vi "get default pixel clock.vi"(8 "error in (no error)":errorcluster, 11 "Thorcam in":refnum<class "Thorcam.lvclass">) -> (0 "error out":errorcluster, 1 "pixel clock":dbl[unit], 3 "Thorcam out":refnum<class "Thorcam.lvclass">)   [LabVIEW 2012, in "Thorcam.lvclass"]
uses:
  Thorcam.lvclass
  Thorcam.lvclass/Thorcam.ctl
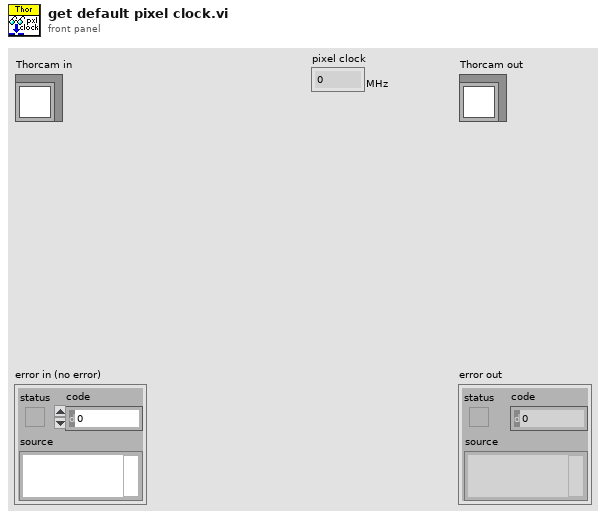
[diagram p1: front panel]
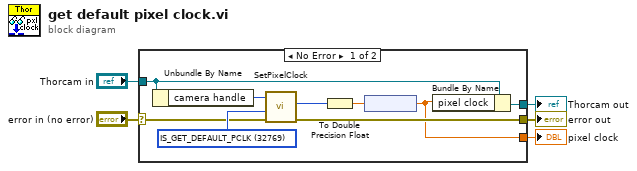
[diagram p0: block diagram]
diagram:
  n1 = case shown="No Error" "error in (no error)" {
    selector: "error in (no error)" -> [w12 w16]
    tunnel: [w11 w16] -> w4
    tunnel: [w9 w15] -> w2
    tunnel: "Thorcam in" -> [w10 w15]
    tunnel: [w8 _] -> w1
    frame No Error {
      w13 = 32769 items=["IS_GET_PIXEL_CLOCK"=32768, "IS_GET_DEFAULT_PCLK"=32769, "IS_SET_PIXEL_CLOCK"=32770] ("Mode")
      n2 = Unbundle By Name(w10) -> ("camera handle"=w7:u32)
      n3 = call <instrlib>:"SetPixelClock.vi"("error in"=w12, "Mode"=w13, "Camera Handle In"=w7) -> ("error out"=w11:errorcluster, "Value"=w14:i32)  [unwired: 6 in, 1 out]
      n4 = To Double Precision Float(number=w14) -> (double precision float=w6:dbl)
      n5 = node(w6) -> (w8:dbl[unit])
      n6 = Bundle By Name(cluster=w10, "pixel clock"=w8) -> (w9:refnum<class "Thorcam.lvclass">)
    }
    frame Error {
    }
  }
  "error out" <- w4
  "Thorcam out" <- w2
  "pixel clock" <- w1
